vi "FTW-JSON-CodeGen-AdaptToInputs.vi"(0 "State In":T1, 5 "XRef":refnum<vi>, 7 "Term Types":cluster{"Type":variant, "ID":string}[](array[cluster])) -> (4 "State Out":T1, 6 "Reply":string[](array[string]))   [LabVIEW 2012, in "FTW-JSON-Deserialize.xnode"]
uses:
  src/JSON/FTW-JSON-Deserialize.xnode
  FTW-JSON-CodeGen-State.ctl
panel:
  # "Inputs"
  # "Outputs"
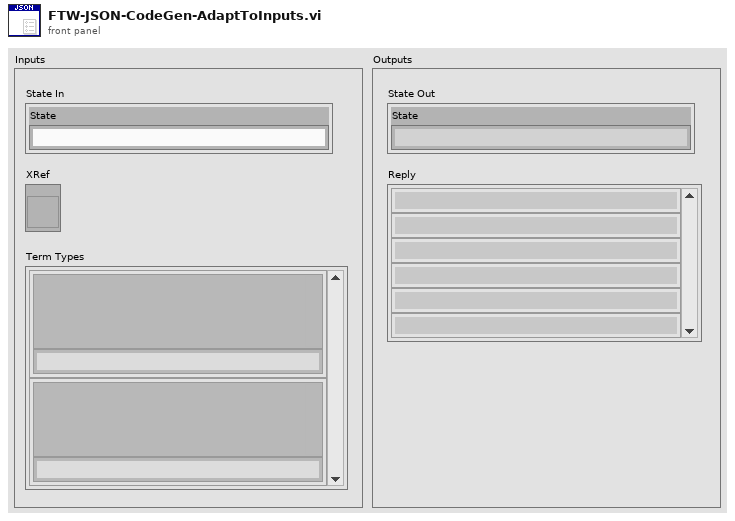
[diagram p1: front panel]
types:
  T1 = typedef "FTW-JSON-Deserialize.xnode/FTW-JSON-CodeGen-State.ctl" = cluster{"State":string}
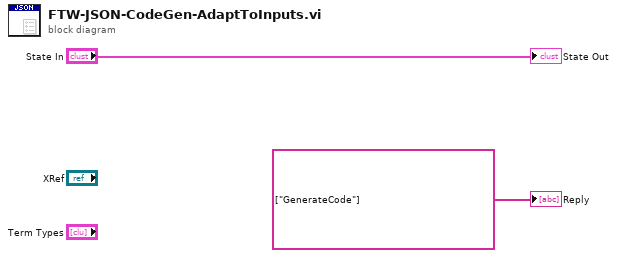
[diagram p0: block diagram]
diagram:
  "State Out" <- "State In"
  "Reply" <- string[] ["GenerateCode"] ("Reply")
